vi "createemptybinary.vi"(8 "base path":path, 9 "file index":u64, 10 "data column":string) -> ()   [LabVIEW 2015]
panel:
  in  "Array":ext[](array[numeric])
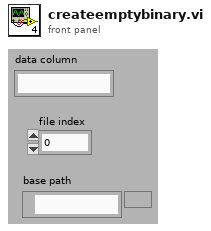
[diagram p1: front panel]
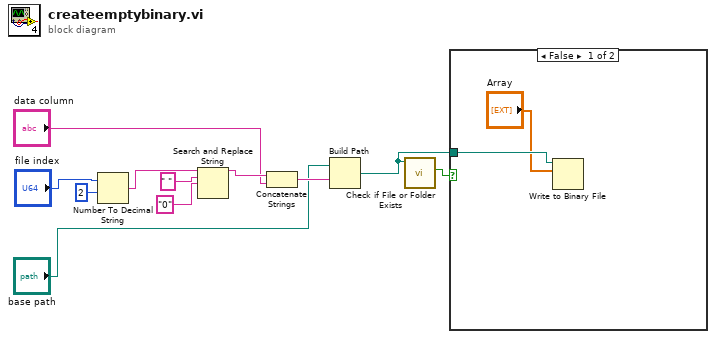
[diagram p0: block diagram]
diagram:
  n1 = Number To Decimal String(number="file index", width (-)=2) -> (decimal integer string=w8:string)
  n2 = Search and Replace String(input string=w8, search string=" ", replace string="0") -> (result string=w7:string)  [unwired: 2 in, 6 out]
  n3 = Concatenate Strings(w7, "data column") -> (w6:string)
  n4 = Build Path(base path="base path", name or relative path=w6) -> (appended path=w1:path)
  n5 = call <vilib>:"Check if File or Folder Exists.vi"("path"=w1) -> ("file or folder exists?"=w2:bool)  [unwired: 1 in, 9 out]
  n6 = case shown="False" w2 {
    tunnel: w1 -> [w13 _]
    frame False {
      n7 = Write to Binary File(file (use dialog)=w13, data="Array") -> ()  [unwired: 1 in, 6 out]
    }
    frame True {
    }
  }
